vi "Generate Firmware Wizard Summary Message.vi"(8 "Error In":errorcluster, 10 "Device ID":u8, 11 "Device Family":T1 items=["National Instruments", "Digilent", "Arduino"]) -> (0 "Error Out":errorcluster, 3 "Summary":string)   [LabVIEW 2011, in "LMH-LINX.lvlib"]
uses:
  LMH-LINX.lvlib
  Type Defs/Device Family.ctl
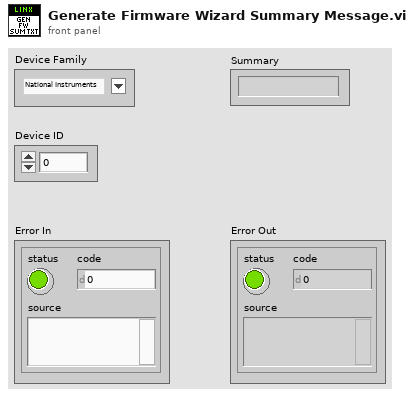
[diagram p1: front panel]
types:
  T1 = typedef "LMH-LINX.lvlib/Device Family.ctl" = u8
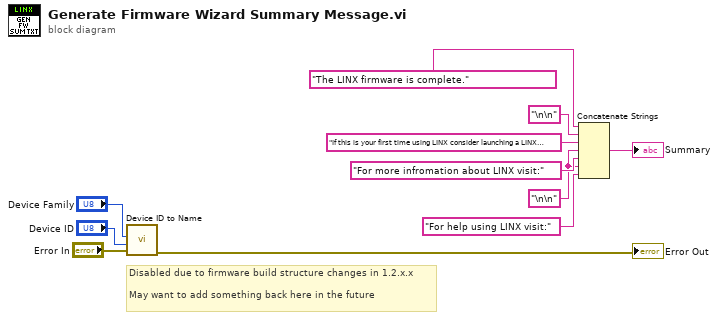
[diagram p0: block diagram]
diagram:
  w4 = "\n\n" ("string")
  # "Disabled due to firmware build structure changes in 1.2.x.x\n\nMay want to add something back here in the future"
  n1 = call "Device ID to Name.vi"("Error In"="Error In", "Device Index"="Device ID", "Family Index"="Device Family") -> ("Error Out"=→"Error Out":errorcluster)  [unwired: 6 in, 2 out]
  n2 = Concatenate Strings("The LINX firmware is complete.", "\n\n" ("string"), "If this is your first time using LINX consider launching a LINX example using the button below.  More LINX examples can befound in the LabVIEW Example Finder by launching LabVIEW and clicking Help>>Find Examples, then searching for 'LINX'." ("string"), w4, "For more infromation about LINX visit:" ("string"), w4, "For help using LINX visit:" ("string")) -> (→"Summary":string)
